vi "MEASURE_hysteresis_multiple_SHG gate.vi"() -> ()   [LabVIEW 2020]
uses:
  <instrlib>/Keithley 24XX/Public/Data/Read (Multiple Points).vi
  <vilib>/Utility/file.llb/Write To Spreadsheet File (DBL).vi
  C/Program Files/National Instruments/LabVIEW 2016/instr.lib/Stanford Research 830/Stanford Research 830.lvlib
  C/Program Files/National Instruments/LabVIEW 2016/instr.lib/Keithley 2450/Keithley 2450.lvlib
  <instrlib>/Keithley 24XX/Keithley 24XX.lvlib
  <vilib>/Analysis/NI_AALBase.lvlib
panel:
  out "XY Graph 2":cluster{dbl[], dbl[]}(graph)
  out "para2 Measurement":dbl
  in  "Parameter2 (1: X)":u16(ring)=1 items=["X"=1, "Y"=2, "R"=3, "Theta"=4, "Channel 1"=5, "Channel 2"=6, "Aux In 1"=7, "Aux In 2"=8, "Aux In 3"=9, "Aux In 4"=10]
  in  "auto phase":bool
  in  "manual phase":dbl
  in  "harm#2":dbl=1.0
  out "top gate leaking":dbl
  out "top gate voltage":dbl format="%#_13g"
  in  "Compliance  Level (1uA)":dbl=2e-08
  in  "Source Mode  (0: Voltage)":u16(ring) items=["Voltage", "Current"]
  in  "top gate thickness":dbl
  in  "bottom gate thickness":dbl
  in  "pure field (T)/pure doping (F)":bool
  in  "Serial Configuration":T1={"Baud Rate"=9600, "Parity"=0, "Data Bits"=8, "Stop Bits"=10, "Flow Control"=0} {"Flow Control" items=["None", "XON/XOFF", "RTS/CTS", "XON/XOFF & RTS/CTS", "DTR/DSR", "XON/XOFF & DTR/DSR"]; "Stop Bits" items=["1.0"=10, "1.5"=15, "2.0"=20]; "Data Bits" items=["7"=7, "8"=8]; "Parity" items=["None", "Odd", "Even", "Mark", "Space"]; "Baud Rate" items=["300"=300, "600"=600, "1200"=1200, "2400"=2400, "4800"=4800, "9600"=9600, "19200"=19200]}
  in  "top gate address":refnum<visa-resource-name>="GPIB0::25::INSTR"
  out "loop run":i32
  in  "loop #":i32
  in  "Save data or not":bool=TRUE
  in  "path (folder + filename)":string="D:\\Kedar\\MoS2\\jw7_DJ_bulk_111213\\VvsHtr\\VvsHtr_300K"
  in  "Clear Plot":bool
  out "XY Graph":cluster{dbl[], dbl[]}(graph)
  out "para1 Measurement":dbl=1.49013e-07
  in  "Parameter (1: X)":u16(ring)=1 items=["X"=1, "Y"=2, "R"=3, "Theta"=4, "Channel 1"=5, "Channel 2"=6, "Aux In 1"=7, "Aux In 2"=8, "Aux In 3"=9, "Aux In 4"=10]
  out "gate voltage":dbl format="%#_13g"
  out "gate leaking":string="defbuffer1"
  in  "GATE STEP(mv)":i32
  in  "GATE Low Value (default 0)":dbl
  in  "GATE High Value":dbl=3.5
  in  "Function (0: Volts) 2":u16(ring) items=["Volts", "Current", "Resistance"]
  in  "Source Compaliance":dbl=1e-08
  in  "back gate address":refnum<visa-resource-name>="GPIB0::18::INSTR"
  in  "SD stabilization(S) 2":dbl=0.1 format="%#_13g"
  in  "Sine Output Amplitude (1 V) 2":dbl=0.05
  in  "GATE / SD stablization 3":dbl=0.1 format="%#_13g"
  in  "frequency":dbl=50.0 format="%#_13g"
  in  "Input Connection (0: Single-Ended Voltage)":u16(ring) items=["Single-Ended Voltage", "Differential Voltage", "1 MOhm Current Gain", "100 MOhm Current Gain"]
  in  "LOCKIN address":refnum<visa-resource-name>="GPIB0::8::INSTR"
  # "Lock-in"
  # "top Gate Setting"
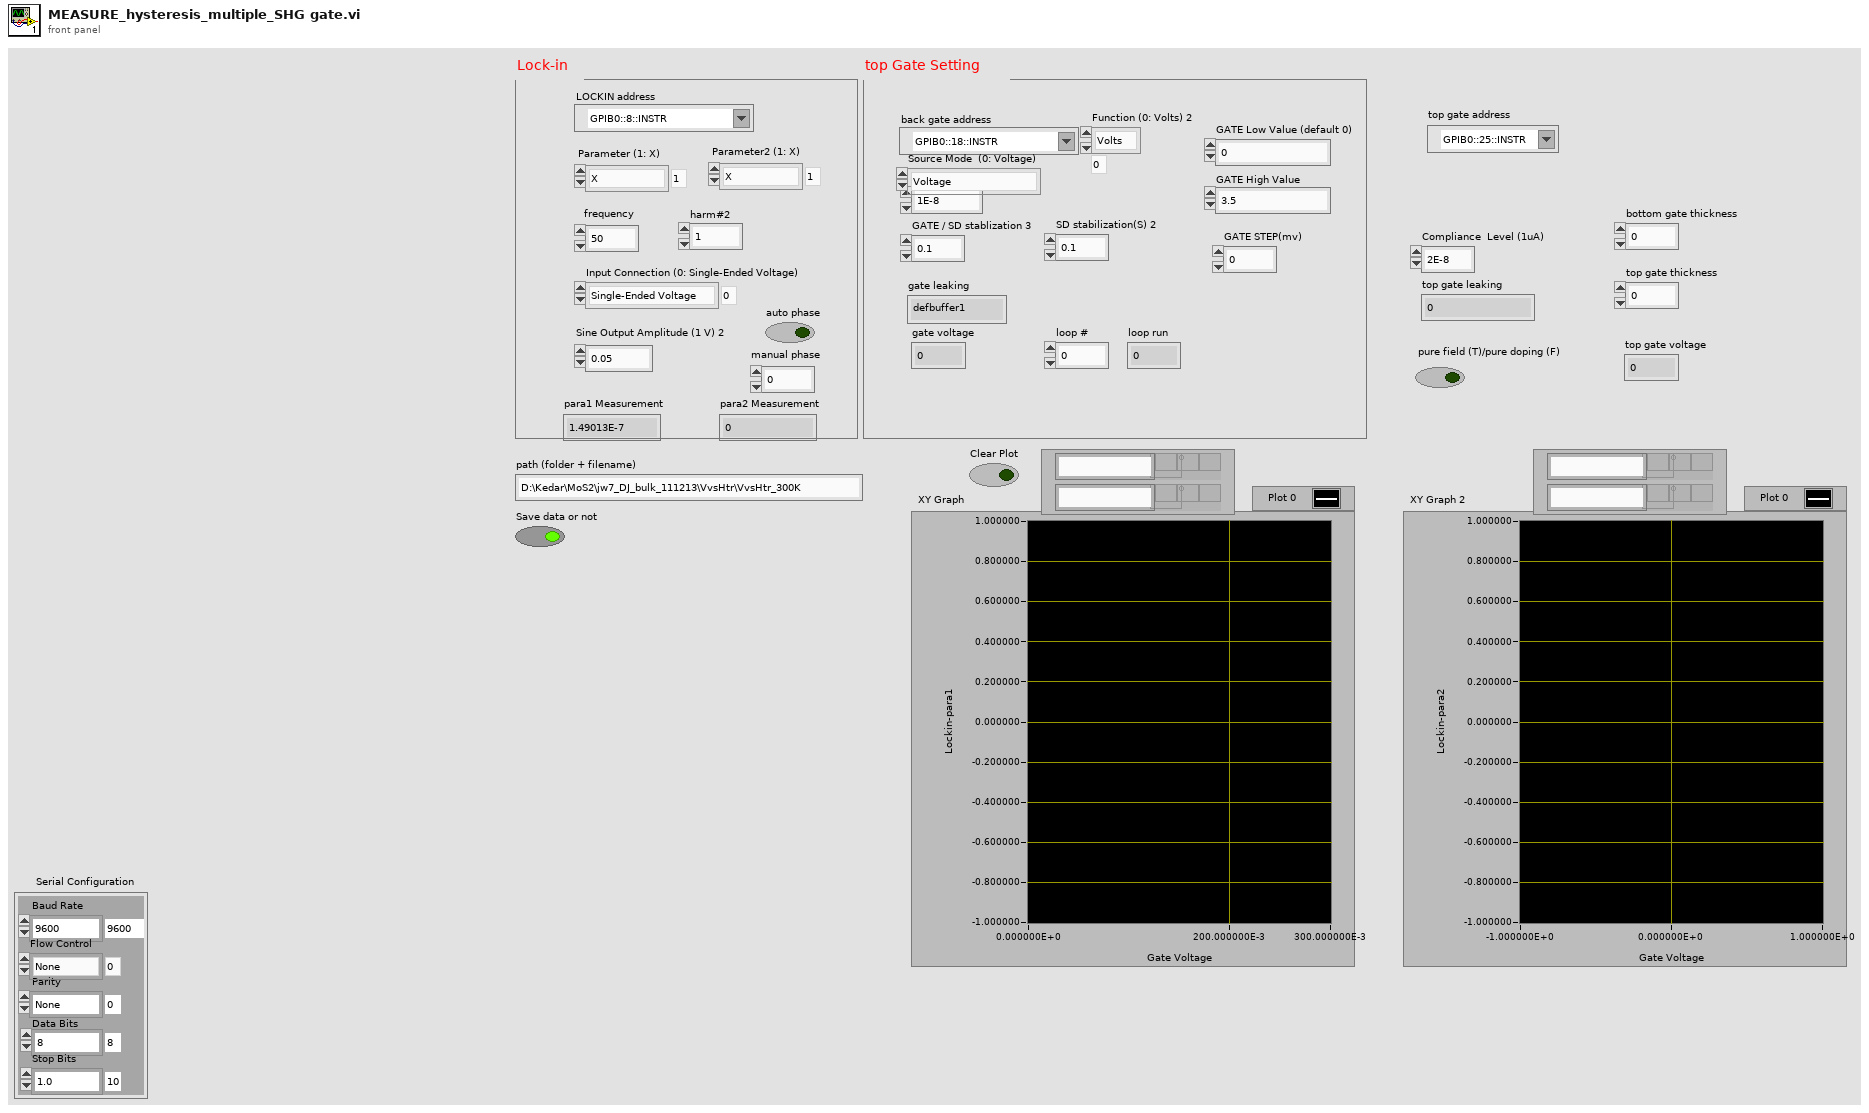
[diagram p1: front panel]
types:
  T1 = cluster{"Baud Rate":u32, "Parity":u16, "Data Bits":u16, "Stop Bits":u16, "Flow Control":u16}
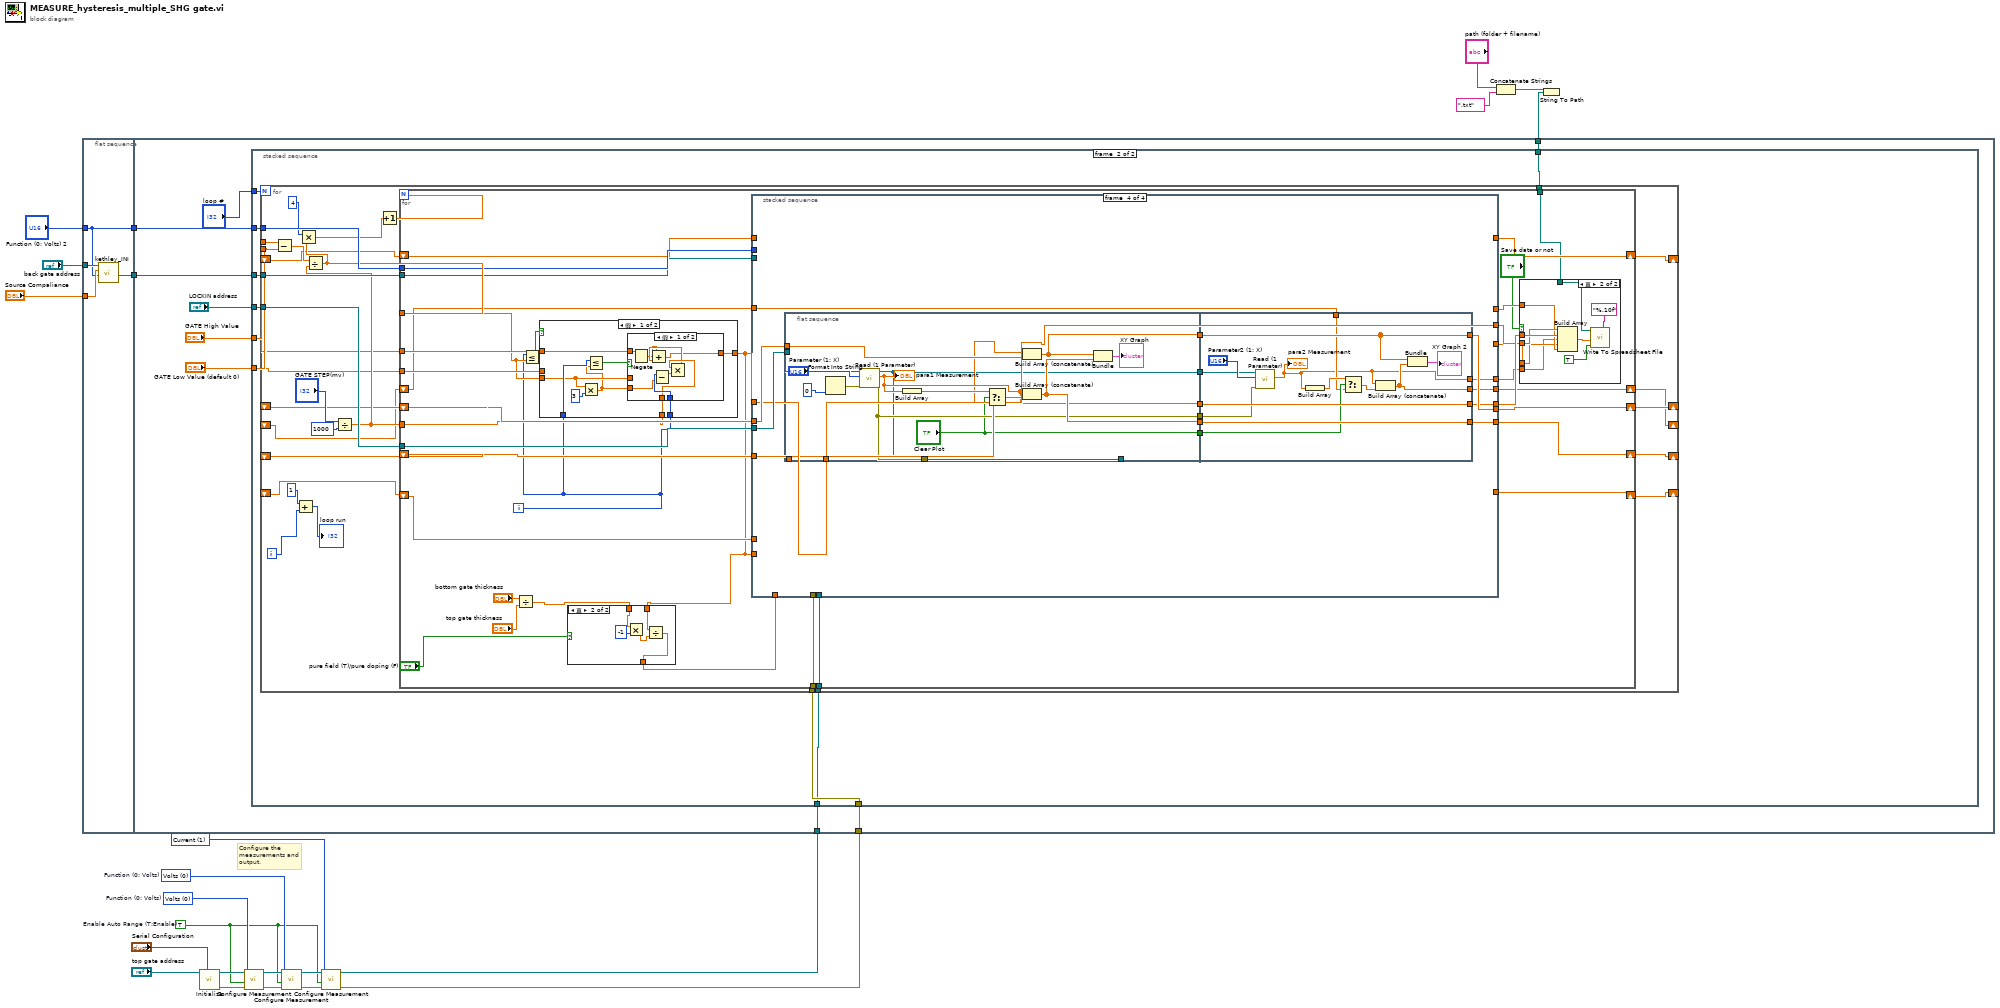
[diagram p0: block diagram]
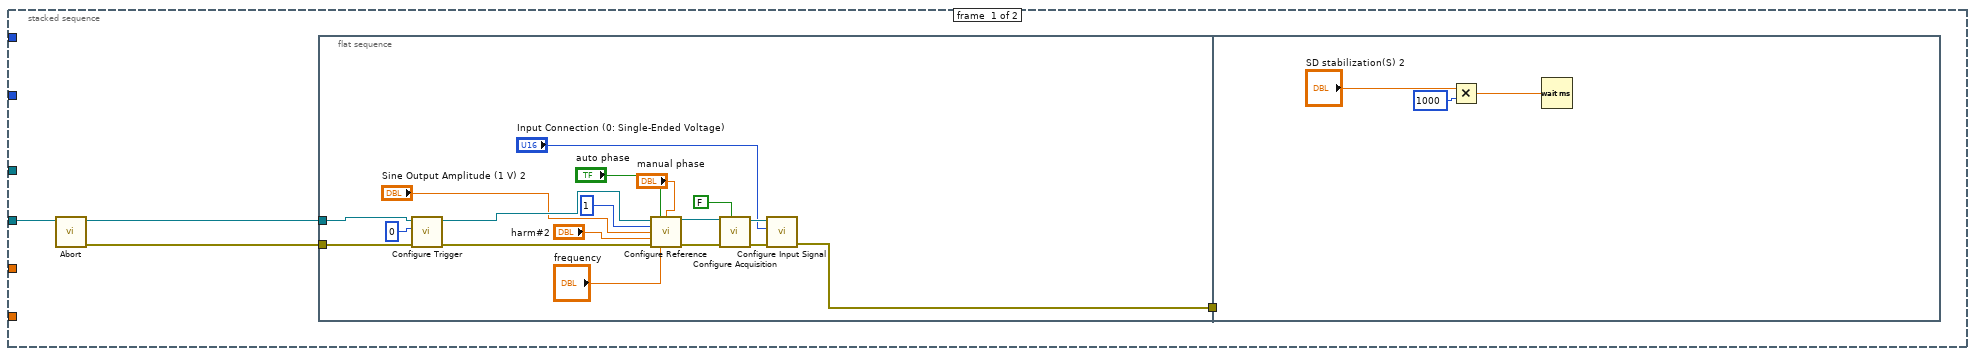
[diagram p2: hidden frame]
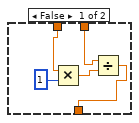
[diagram p3: hidden frame]
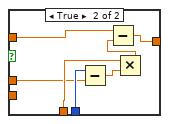
[diagram p5: hidden frame]
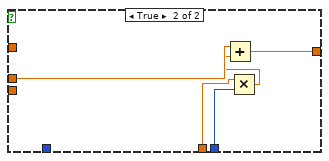
[diagram p6: hidden frame]
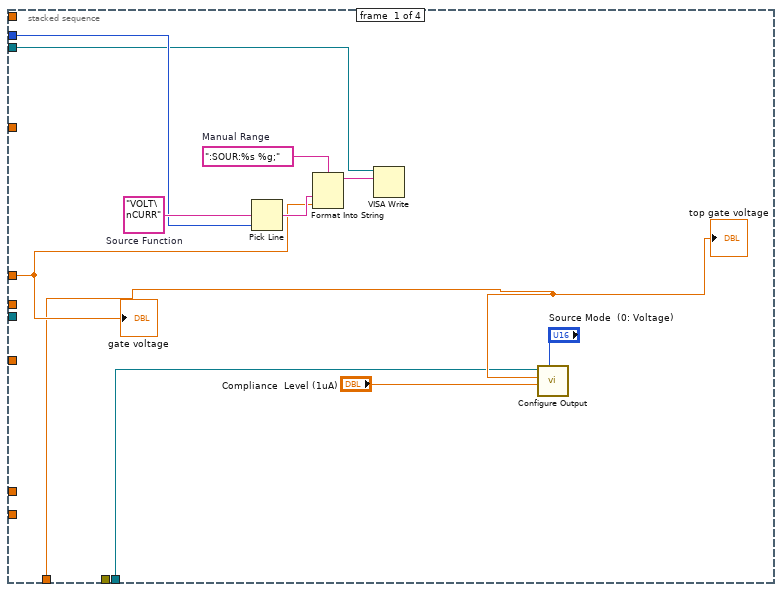
[diagram p7: hidden frame]
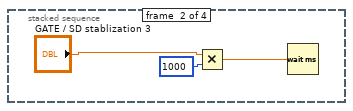
[diagram p8: hidden frame]
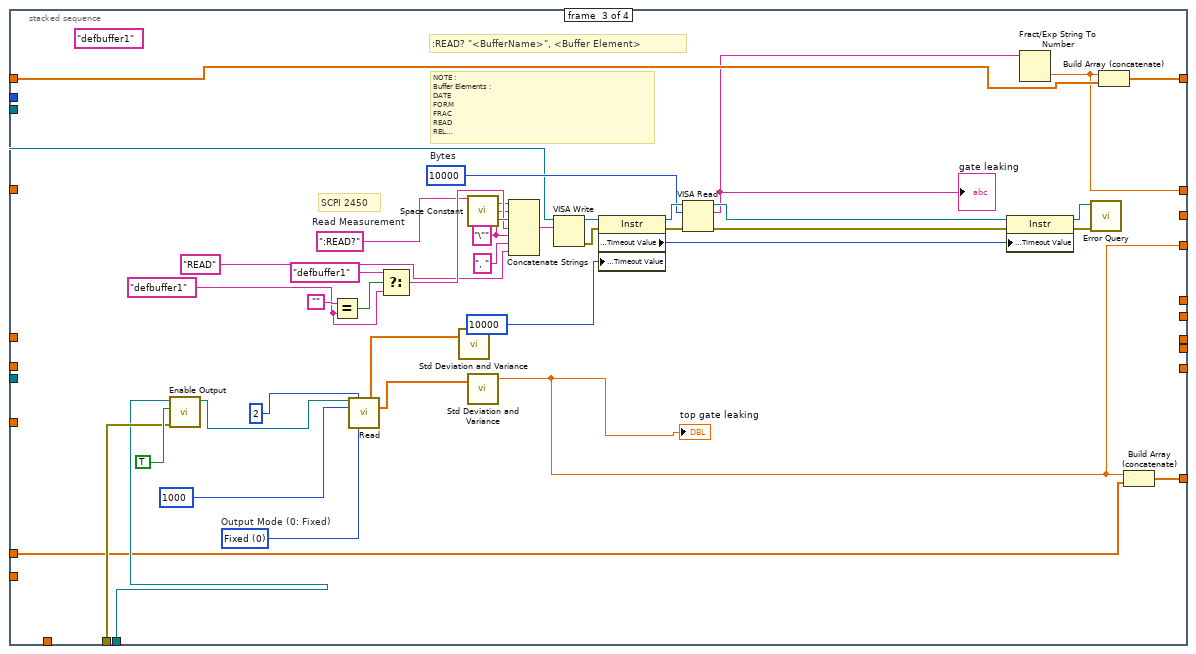
[diagram p9: hidden frame]
diagram:
  w3 = u16 1 items=["Volts", "Current", "Resistance"] ("Function (0: Volts)")
  w4 = TRUE  # Enable Auto Range (T:Enable)
  w7 = u16 0 items=["Volts", "Current", "Resistance"]  # Function (0: Volts)
  w8 = u16 0 items=["Volts", "Current", "Resistance"]  # Function (0: Volts)
  # "Configure the measurements and output."
  n1 = flat-sequence {
    tunnel: "back gate address" -> [w27]
    tunnel: "Source Compaliance" -> [w26]
    tunnel: "Function (0: Volts) 2" -> [w24]
    tunnel: [w25] -> w20
    tunnel: [w24] -> w19
    tunnel: w20 -> [w35]
    tunnel: w19 -> [w34]
    tunnel: w15 -> [w31]
    tunnel: w2 -> [w29]
    tunnel: w1 -> [w28]
    frame #0 {
      n2 = call "kethley_INI.vi"("Function (0: Volts) in"=w24, "Source Compaliance"=w26, "VISA Refnum in"=w27) -> ("VISA resource name out"=w25:refnum<visa-resource-name>)  [unwired: 8 in]
    }
    frame #1 {
      n3 = stacked-sequence {
        tunnel: "LOCKIN address" -> [w39 w68]
        tunnel: w35 -> [_ w69]
        tunnel: w34 -> [_ w70]
        tunnel: "GATE High Value" -> [_ w66]
        tunnel: "GATE Low Value (default 0)" -> [_ w67]
        tunnel: w31 -> [_ w65]
        tunnel: "loop #" -> [_ w64]
        tunnel: w29 -> [_ w62]
        tunnel: w28 -> [_ w63]
        frame #0 {
          n4 = call "Abort.vi"("VISA resource name"=w39) -> ("error out"=w37:errorcluster, "VISA resource name out"=w38:refnum<visa-resource-name>)  [unwired: 9 in]
          n5 = flat-sequence {
            tunnel: w38 -> [w58]
            tunnel: [w43] -> w40
            tunnel: w37 -> [w42]
            tunnel: w40 -> [_]
            frame #0 {
              n6 = call "Configure Trigger.vi"("error in (no error)"=w42, "Trigger Source (0: Internal)"=0, "VISA resource name"=w58) -> ("error out"=w52:errorcluster, "VISA resource name out"=w53:refnum<visa-resource-name>)  [unwired: 7 in]
              n7 = call "Configure Reference.vi"("VISA resource name"=w53, "Auto Phase (T: Enabled)"="auto phase", "Manual Phase (0 Degree)"="manual phase", "Reference Source (1: Internal)"=1, "Sine Output Amplitude (1 V)"="Sine Output Amplitude (1 V) 2", "Detection Harmonic Number (1)"="harm#2", "error in (no error)"=w52, "Internal Reference Frequency (1000 Hz)"="frequency") -> ("VISA resource name out"=w50:refnum<visa-resource-name>, "error out"=w45:errorcluster)  [unwired: 6 in]
              n8 = call "Configure Acquisition.vi"("Continuous Storage (T: Enable)"=FALSE, "error in (no error)"=w45, "VISA resource name"=w50) -> ("error out"=w44:errorcluster, "VISA resource name out"=w48:refnum<visa-resource-name>)  [unwired: 7 in]
              n9 = call "Configure Input Signal.vi"("error in (no error)"=w44, "Input Connection (0: Single-Ended Voltage)"="Input Connection (0: Single-Ended Voltage)", "VISA resource name"=w48) -> ("error out"=w43:errorcluster)  [unwired: 7 in, 1 out]
            }
            frame #1 {
              n10 = Multiply(x="SD stabilization(S) 2", y=1000) -> (x*y=w61:dbl)
              n11 = Wait (ms)(milliseconds to wait=w61) -> ()  [unwired: 1 out]
            }
          }
        }
        frame #1 {
          n12 = for {
            N: w64 -> [_]
            tunnel: w70 -> [w99]
            tunnel: w69 -> [w98]
            tunnel: w68 -> [w97]
            tunnel: w67 -> [w91]
            tunnel: w66 -> [w90]
            tunnel: w65 -> [w89]
            shift-right: [w85] -> _
            shift-left: _ -> [w84]
            shift-right: [w83] -> _
            shift-left: _ -> [w81]
            shift-right: [w82] -> _
            shift-left: _ -> [w80]
            tunnel: w63 -> [w76]
            tunnel: w62 -> [w75]
            shift-right: [w74] -> _
            shift-left: _ -> [w73]
            shift-right: [w72] -> _
            shift-left: _ -> [w71]
            i -> [w78]
            n13 = Subtract(x=w90, y=w91) -> (x-y=w93:dbl)
            n14 = Add(x=1, y=w78) -> (x+y=→"loop run":i32)
            n15 = Divide(x="GATE STEP(mv)", y=1000) -> (x/y=w92:dbl)
            n16 = Divide(x=w93, y=w92) -> (x/y=w88:dbl)
            n17 = Multiply(x=4, y=w88) -> (x*y=w87:dbl)
            n18 = Increment(x=w87) -> (x+1=w86:dbl)
            n19 = for {
              N: w86 -> [_]
              tunnel: w99 -> [w133]
              tunnel: w98 -> [w132]
              tunnel: w97 -> [w131]
              tunnel: w92 -> [w122]
              shift-right: [w130] -> w85
              shift-left: w84 -> [w129]
              shift-right: [w126] -> w82
              shift-left: w80 -> [w128]
              shift-right: [w125] -> w83
              shift-left: w81 -> [w127]
              tunnel: w88 -> [w120]
              tunnel: w91 -> [w123]
              tunnel: w90 -> [w121]
              tunnel: w89 -> [w115]
              tunnel: w76 -> [w108]
              tunnel: w75 -> [w107]
              shift-right: [w106] -> w74
              shift-left: w73 -> [w105]
              shift-right: [w102] -> w72
              shift-left: w71 -> [w101]
              i -> [w119]
              n20 = Divide(x="bottom gate thickness", y="top gate thickness") -> (x/y=w113:dbl)
              n21 = Less Or Equal?(x=w119, y=w120) -> (x <= y?=w124:bool)
              n22 = case shown="假" w124 {
                tunnel: w123 -> [_ w181]
                tunnel: w119 -> [w161 w180]
                tunnel: w122 -> [w160 w179]
                tunnel: [w158 w177] -> w103
                tunnel: w121 -> [w159 _]
                tunnel: w120 -> [w154 _]
                tunnel: w119 -> [w157 _]
                frame False {
                  n23 = Multiply(x=w154, y=3) -> (x*y=w153:dbl)
                  n24 = Less Or Equal?(x=w157, y=w153) -> (x <= y?=w155:bool)
                  n25 = case shown="假" w155 {
                    tunnel: w161 -> [w169 w176]
                    tunnel: w160 -> [w167 w174]
                    tunnel: w159 -> [w163 w172]
                    tunnel: [w165 w171] -> w158
                    tunnel: w154 -> [_ w170]
                    tunnel: w153 -> [w162 _]
                    frame False {
                      n26 = Negate(x=w163) -> (-x=w164:dbl)
                      n27 = Subtract(x=w169, y=w162) -> (x-y=w168:dbl)
                      n28 = Multiply(x=w167, y=w168) -> (x*y=w166:dbl)
                      n29 = Add(x=w164, y=w166) -> (x+y=w165:dbl)
                    }
                    frame True {
                      n30 = Subtract(x=w176, y=w170) -> (x-y=w175:dbl)
                      n31 = Multiply(x=w174, y=w175) -> (x*y=w173:dbl)
                      n32 = Subtract(x=w172, y=w173) -> (x-y=w171:dbl)
                    }
                  }
                }
                frame True {
                  n33 = Multiply(x=w179, y=w180) -> (x*y=w178:dbl)
                  n34 = Add(x=w181, y=w178) -> (x+y=w177:dbl)
                }
              }
              n35 = case shown="真" "pure field (T)/pure doping (F)" {
                tunnel: w113 -> [w137 w143]
                tunnel: [w134 w141] -> w109
                tunnel: w103 -> [w135 w140]
                frame False {
                  n36 = Multiply(x=w137, y=1) -> (x*y=w136:dbl)
                  n37 = Divide(x=w135, y=w136) -> (x/y=w134:dbl)
                }
                frame True {
                  n38 = Multiply(x=w143, y=-1) -> (x*y=w139:dbl)
                  n39 = Divide(x=w140, y=w139) -> (x/y=w141:dbl)
                }
              }
              n40 = stacked-sequence {
                tunnel: w133 -> [w188 _ _ _]
                tunnel: w132 -> [w187 _ w212 _]
                tunnel: w131 -> [_ _ _ w246]
                tunnel: w103 -> [w186 _ _ w244]
                tunnel: [_ _ w210 _] -> w130
                tunnel: w129 -> [_ _ w211 _]
                tunnel: w128 -> [_ _ _ w250]
                tunnel: w127 -> [_ _ _ w247]
                tunnel: [_ _ _ w249] -> w126
                tunnel: [_ _ _ w248] -> w125
                tunnel: [_ _ _ w245] -> w118
                tunnel: [_ _ _ w244] -> w117
                tunnel: [_ _ w208 _] -> w116
                tunnel: w109 -> [w183 _ _ _]
                tunnel: w108 -> [_ _ w200 _]
                tunnel: w107 -> [w182 _ w199 _]
                tunnel: [_ _ w198 _] -> w106
                tunnel: w105 -> [_ _ w197 _]
                tunnel: [_ _ w196 _] -> w104
                tunnel: w103 -> [_ _ _ _]
                tunnel: [_ _ _ w237] -> w102
                tunnel: w101 -> [_ _ _ w236]
                tunnel: [_ _ _ w235] -> w100
                frame #0 {
                  w190 = "VOLT\nCURR"  # Source Function
                  w191 = ":SOUR:%s %g;"  # Manual Range
                  n41 = Pick Line(multi-line string=w190, line index=w188) -> (output string=w189:string)  [unwired: 1 out]
                  n42 = Format Into String(format string=w191, w189, w186) -> (resulting string=w192:string)  [unwired: 2 in, 1 out]
                  n43 = VISA Write(VISA resource name=w187, write buffer=w192) -> ()  [unwired: 1 in, 3 out]
                  n44 = call <instrlib>:"Configure Output.vi"("Source Mode  (0: Voltage)"="Source Mode  (0: Voltage)", "Compliance  Level (0.1)"="Compliance  Level (1uA)", "Output Level (0)"=w183, "VISA resource name"=w182) -> ()  [unwired: 6 in, 2 out]
                  "gate voltage" <- w186
                  "top gate voltage" <- w183
                }
                frame #1 {
                  n45 = Multiply(x="GATE / SD stablization 3", y=1000) -> (x*y=w195:dbl)
                  n46 = Wait (ms)(milliseconds to wait=w195) -> ()  [unwired: 1 out]
                }
                frame #2 {
                  w205 = u16 0 items=["Fixed", "Sweep", "List"]  # Output Mode (0: Fixed)
                  w223 = "defbuffer1" ("Buffer Name (defbuffer1) 2")
                  (unwired) "defbuffer1" ("t")
                  w221 = "\""
                  w218 = ":READ?"  # Read Measurement
                  w227 = u32 10000  # Bytes
                  # "NOTE :\nBuffer Elements :\nDATE\nFORM\nFRAC\nREAD\nREL\nSEC\nSOUR\nSOURFORM\nSOURSTAT\nSOURUNIT\nSTAT\nTIME\nTsT\nUNIT"
                  # ":READ? \"<BufferName>\", <Buffer Element>"
                  # "SCPI 2450"
                  n47 = call <instrlib>:"Enable Output.vi"("error in (no error)"=w200, "Enable Output (T: Enable)"=TRUE, "VISA resource name"=w199) -> ("VISA resource name out"=w201:refnum<visa-resource-name>)  [unwired: 7 in, 1 out]
                  n48 = Equal?(x="", y=w223) -> (x = y?=w224:bool)
                  n49 = call-poly <instrlib>:"Read.vi"("VISA resource name"=w201, "Sample Count (1)"=u32 2 ("Number of Samples"), "Timeout (10000 ms)"=1000, "Output Mode (0: Fixed)"=w205) -> ("Voltage"=w203:sgl[], "Current"=w204:sgl[])  [unwired: 5 in, 5 out]
                  n50 = Select(t="defbuffer1", s=w224, f=w223) -> (s? t:f=w220:string)
                  n51 = call <vilib>:"Std Deviation and Variance.vi"("X"=w203) -> ()  [unwired: 1 in, 3 out]
                  n52 = call <vilib>:"Space Constant.vi"() -> ("String"=w219:string)
                  n53 = call <vilib>:"Std Deviation and Variance.vi"("X"=w204) -> ("mean"=w196:dbl)  [unwired: 1 in, 2 out]
                  "top gate leaking" <- w196
                  n54 = Concatenate Strings(w218, w219, w221, w220, w221, ", " ("string"), "READ" ("Buffer Elements 2")) -> (w234:string)
                  n55 = VISA Write(VISA resource name=w212, write buffer=w234) -> (VISA resource name out=w226:refnum<visa-resource-name>, error out=w233:errorcluster)  [unwired: 1 in, 1 out]
                  n56 = property class="Instr"(reference=w226, error in=w233, "General Settings:Timeout Value"=10000 ("Timeout (10000 ms) 2")) -> (reference out=w232:refnum<visa-resource-name>, error out=w231:errorcluster, "General Settings:Timeout Value"=w228:u32)
                  n57 = VISA Read(VISA resource name=w232, byte count=w227, error in (no error)=w231) -> (VISA resource name out=w230:refnum<visa-resource-name>, read buffer=w209:string, error out=w229:errorcluster)  [unwired: 1 out]
                  "gate leaking" <- w209
                  n58 = property class="Instr"(reference=w230, error in=w229, "General Settings:Timeout Value"=w228) -> (reference out=w216:refnum<visa-resource-name>, error out=w215:errorcluster)
                  n59 = Fract/Exp String To Number(string=w209) -> (number=w208:dbl)  [unwired: 3 in, 1 out]
                  n60 = call "Error Query.vi"("error in (no error)"=w215, "VISA resource name"=w216) -> ()  [unwired: 10 out]
                  n61 = Build Array (concatenate)(w208, w211) -> (w210:dbl[])
                  n62 = Build Array (concatenate)(w196, w197) -> (w198:dbl[])
                }
                frame #3 {
                  n63 = flat-sequence {
                    tunnel: w250 -> [w260]
                    tunnel: w247 -> [w257]
                    tunnel: w246 -> [w256]
                    tunnel: w244 -> [w254]
                    tunnel: [w252] -> _
                    tunnel: [w253] -> _
                    tunnel: [w259] -> w243
                    tunnel: [w258] -> w242
                    tunnel: [w255] -> w241
                    tunnel: [w253] -> w240
                    tunnel: [w252] -> w239
                    tunnel: ["Clear Plot"] -> w238
                    tunnel: [w278] -> w245
                    tunnel: [w272] -> w248
                    tunnel: [w279] -> w249
                    tunnel: w243 -> [w279]
                    tunnel: w242 -> [w272]
                    tunnel: w241 -> [w278]
                    tunnel: w240 -> [w276]
                    tunnel: w239 -> [w275]
                    tunnel: w238 -> [w273]
                    tunnel: [w270] -> w237
                    tunnel: w236 -> [w269]
                    tunnel: [w267] -> w235
                    frame #0 {
                      n64 = Format Into String(0) -> (error out=w266:errorcluster)  [unwired: 3 in, 1 out]
                      n65 = call "Read (1 Parameter).vi"("error in (no error)"=w266, "Parameter (1: X)"="Parameter (1: X)", "VISA resource name"=w256) -> ("error out"=w253:errorcluster, "Measurement"=w255:dbl, "VISA resource name out"=w252:refnum<visa-resource-name>)  [unwired: 6 in]
                      "para1 Measurement" <- w255
                      n66 = Build Array(w255) -> (w263:dbl[])
                      n67 = Select(t=w263, s="Clear Plot", f=w260) -> (s? t:f=w264:dbl[])
                      n68 = Build Array (concatenate)(w254, w257) -> (w258:dbl[])
                      n69 = Build Array (concatenate)(w255, w264) -> (w259:dbl[])
                      n70 = Bundle(w258, w259) -> (→"XY Graph":cluster{dbl[], dbl[]})  [unwired: 1 in]
                    }
                    frame #1 {
                      n71 = call "Read (1 Parameter).vi"("error in (no error)"=w276, "Parameter (1: X)"="Parameter2 (1: X)", "VISA resource name"=w275) -> ("Measurement"=w267:dbl)  [unwired: 6 in, 2 out]
                      "para2 Measurement" <- w267
                      n72 = Build Array(w267) -> (w274:dbl[])
                      n73 = Select(t=w274, s=w273, f=w269) -> (s? t:f=w271:dbl[])
                      n74 = Build Array (concatenate)(w267, w271) -> (w270:dbl[])
                      n75 = Bundle(w272, w270) -> (→"XY Graph 2":cluster{dbl[], dbl[]})  [unwired: 1 in]
                    }
                  }
                }
              }
              n76 = case shown="真" "Save data or not" {
                tunnel: w118 -> [_ w152]
                tunnel: w117 -> [_ w151]
                tunnel: w116 -> [_ w150]
                tunnel: w115 -> [_ w148]
                tunnel: w104 -> [_ w145]
                tunnel: w100 -> [_ w144]
                frame False {
                }
                frame True {
                  n77 = Build Array(w151, w152, w144, w145, w150) -> (w149:dbl[])
                  n78 = call-poly <vilib>:"Write To Spreadsheet File.vi"("format (%.3f)"="%.10f", "append to file? (new file:F)"=TRUE, "1D data"=w149, "file path (dialog if empty)"=w148) -> ()  [unwired: 4 in, 1 out]
                }
              }
            }
          }
        }
      }
    }
  }
  n79 = call <instrlib>:"Initialize.vi"("Serial Configuration"="Serial Configuration", "VISA resource name"="top gate address") -> ("error out"=w13:errorcluster, "VISA resource name out"=w14:refnum<visa-resource-name>)  [unwired: 8 in]
  n80 = call <instrlib>:"Configure Measurement.vi"("error in (no error)"=w13, "Enable Auto Range (T:Enable)"=w4, "Function (0: Volts)"=w8, "VISA resource name"=w14) -> ("error out"=w12:errorcluster, "VISA resource name out"=w11:refnum<visa-resource-name>)  [unwired: 6 in]
  n81 = call <instrlib>:"Configure Measurement.vi"("error in (no error)"=w12, "Enable Auto Range (T:Enable)"=w4, "Function (0: Volts)"=w7, "VISA resource name"=w11) -> ("error out"=w5:errorcluster, "VISA resource name out"=w6:refnum<visa-resource-name>)  [unwired: 6 in]
  n82 = call <instrlib>:"Configure Measurement.vi"("error in (no error)"=w5, "Enable Auto Range (T:Enable)"=w4, "Function (0: Volts)"=w3, "VISA resource name"=w6) -> ("error out"=w1:errorcluster, "VISA resource name out"=w2:refnum<visa-resource-name>)  [unwired: 6 in]
  n83 = Concatenate Strings("path (folder + filename)", ".txt") -> (w16:string)
  n84 = String To Path(string=w16) -> (path=w15:path)
